vi "test-json-schema-recursive-defs.vi"() -> ()   [LabVIEW 2019, in "TEST-JSON-Schema.lvlib"]
uses:
  TEST-JSON-Schema.lvlib
  typedefs/test_cluster--cluster.ctl
  typedefs/test_enum--enum.ctl
  typedefs/test_nested_cluster--cluster.ctl
  JSON-Schema/JSON-Schema.lvlib
  <vilib>/JDP Science/JSONtext/JSONtext.lvlib
  <vilib>/Utility/Data Type/NI_Data Type.lvlib
panel:
  in  "test object":enum16{"enum", "cluster", "nested cluster"}(ring)
  out "control name|filename":string[](array[string])
  out "JSON Schema out":string
  out "Typedef?":bool[](array[boolean])
  out "JSON Schema out":string
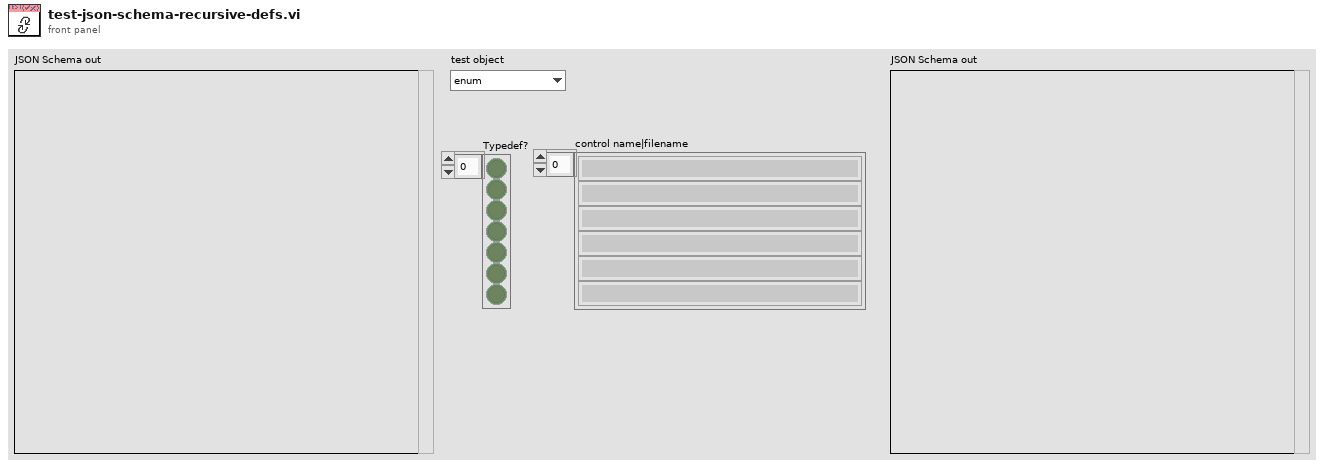
[diagram p1: front panel]
types:
  T1 = typedef "TEST-JSON-Schema.lvlib/test_cluster--cluster.ctl" = cluster{"numeric":dbl, "test_enum":T2}
  T2 = typedef "TEST-JSON-Schema.lvlib/test_enum--enum.ctl" = enum16{"option_1", "option_2"}
  T3 = typedef "TEST-JSON-Schema.lvlib/test_nested_cluster--cluster.ctl" = cluster{"string":string, "test_cluster":T1}
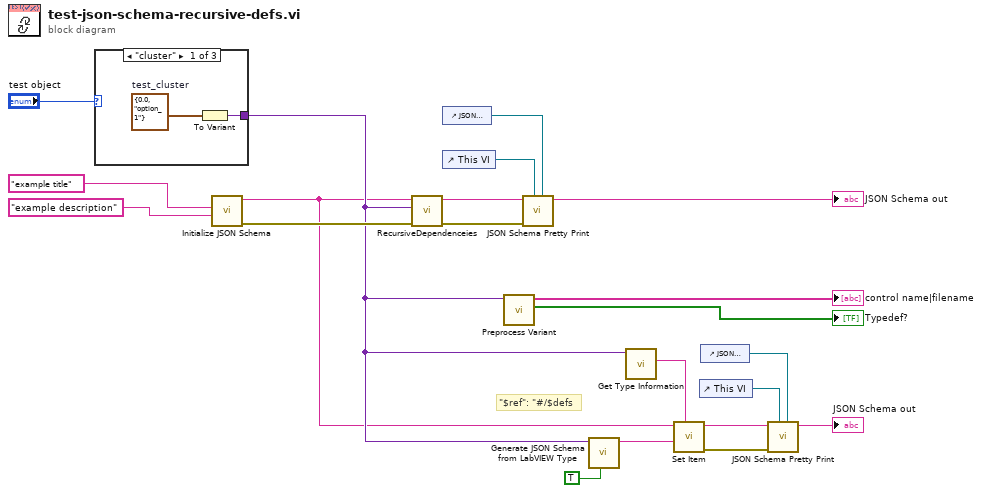
[diagram p0: block diagram]
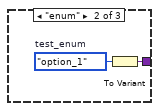
[diagram p2: hidden frame]
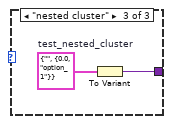
[diagram p3: hidden frame]
diagram:
  # "\"$ref\": \"#/$defs"
  n1 = case shown="\"cluster\"" "test object" {
    tunnel: [w22 w24 w26] -> w12
    frame "cluster" {
      w23 = T1 {"numeric"=0.0, "test_enum"=enum."option_1"}  # test_cluster
      n2 = To Variant(anything=w23) -> (Variant=w22:variant)
    }
    frame "enum" {
      w25 = test_enum--enum."option_1"  # test_enum
      n3 = To Variant(anything=w25) -> (Variant=w24:variant)
    }
    frame "nested cluster" {
      w27 = T3 {"string"="", "test_cluster"={"numeric"=0.0, "test_enum"=enum."option_1"}}  # test_nested_cluster
      n4 = To Variant(anything=w27) -> (Variant=w26:variant)
    }
  }
  n5 = call "Initialize JSON Schema.vi"("Description"="example description", "Title"="example title") -> ("error out"=w21:errorcluster, "JSON Schema out"=w1:string)  [unwired: 8 in]
  n6 = call "RecursiveDependenceies.vi"("error in (no error)"=w21, "Object"=w12, "JSON Schema in"=w1) -> ("error out"=w11:errorcluster, "JSON Schema out"=w10:string)  [unwired: 7 in]
  n7 = control-ref of="JSON Schema out"() -> (w8:refnum<vi>)
  n8 = control-ref of="This VI"() -> (w9:refnum<vi>)
  n9 = call "Preprocess Variant.vi"("Variant"=w12) -> ("typedef?"=→"Typedef?":bool[], "name|filename"=→"control name|filename":string[])  [unwired: 9 in]
  n10 = call "JSON Schema Pretty Print.vi"("String Control"=w8, "reference"=w9, "error in (no error)"=w11, "<JSON> in"=w10) -> ("<JSON> out"=→"JSON Schema out":string)  [unwired: 6 in, 1 out]
  n11 = call <vilib>:"Generate JSON Schema from LabVIEW Type.vi"("Strict Clusters"=TRUE, "Variant"=w12) -> ("JSON Schema"=w16:string)  [unwired: 8 in, 1 out]
  n12 = call <vilib>:"Get Type Information.vi"("variant"=w12) -> ("name"=w17:string)  [unwired: 6 in, 4 out]
  n13 = call <vilib>:"Set Item.vi"("$Path or Item Name"=w17, "JSON to Insert"=w16, "JSON"=w1) -> ("error out"=w2:errorcluster, "<JSON>"=w6:string)  [unwired: 5 in, 1 out]
  n14 = control-ref of="This VI"() -> (w3:refnum<vi>)
  n15 = control-ref of="JSON Schema out"() -> (w4:refnum<vi>)
  n16 = call "JSON Schema Pretty Print.vi"("String Control"=w4, "reference"=w3, "error in (no error)"=w2, "<JSON> in"=w6) -> ("<JSON> out"=→"JSON Schema out":string)  [unwired: 6 in, 1 out]
